vi "Robot Global Data.vi"() -> ()   [LabVIEW 2012]
doc: "This global VI can contain as many global variables as you need. Place a control on the panel, give it a good name. To read or write to it from a VI, drag the icon to the diagram of that VI. You can also drag from the project. Click on the node to change which global you access. You shouldn't have multiple locations writing to a global or it will cause a race-condition."
uses:
  <vilib>/Rock Robotics/WPI/Camera/WPI_CameraImageSize.ctl
  <vilib>/Rock Robotics/WPI/DriverStation/WPI_DriverStationRobotMode2.ctl
panel:
  in  "Angle Setpoint":dbl
  in  "Lower Angle Limit":dbl=0.3
  in  "Upper Angle Limit":dbl=9.7
  in  "Stow Value":dbl
  in  "Shooter motor 2 speed":dbl=1.0
  in  "Shooter motor 1 speed":dbl=1.0
  in  "Ball Release Delay in Milliseconds":i32=250
  in  "Delay after Ball is Release":u32=250
  in  "Delay in Milliseconds":i32=250
  in  "Drive Motor Scale":dbl=100.0
  in  "Numeric 6":dbl
  in  "Numeric 5":dbl
  in  "Numeric 4":dbl
  in  "Numeric 3":dbl
  in  "Numeric 2":dbl
  in  "Numeric 1":dbl
  in  "Robot Mode":T1=enum."Finish"
  in  "LED toggle rate (ms)":u32=100
  in  "image size":T2=enum."320x240"
  in  "Enable Vision":bool
  # "1000 Milliseconds = 1 Second"
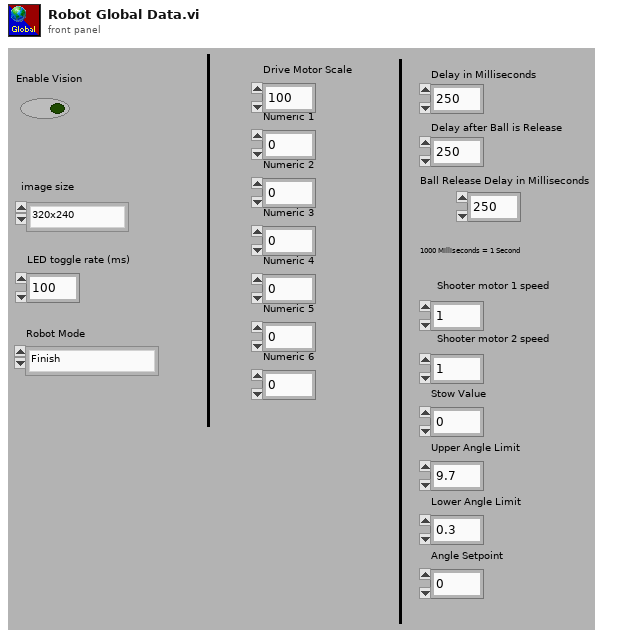
[diagram p1: front panel]
types:
  T1 = typedef "WPI_DriverStationRobotMode2.ctl" = enum16{"Autonomous Disabled", "Autonomous Enabled", "Teleop Disabled", "Teleop Enabled", "Timeout", "Finish", "Test Disabled", "Test Enabled"}
  T2 = typedef "WPI_CameraImageSize.ctl" = enum16{"640x480", "320x240", "160x120"}
diagram:
